vi "DOCK_REPORT_CBATCH_listbox_set_values_and_recolor.vi"(7 "column_names":string[](array[string]), 8 "error_in":errorcluster, 11 "REPORT_all_info_in":T1) -> (0 "error_out":errorcluster, 3 "REPORT_all_info_out":T1)   [LabVIEW 2019]
uses:
  FGV/DOCK_REPORT_records_display/DOCK_REPORT_all_info.ctl
  SQL_CLIENT/MAIN/REPORTS/DATES/typedef/REPORT_DATES_statuses.ctl
  FGV/DOCK_REPORT_records_display/DOCK_REPORT_references.ctl
  <vilib>/Utility/miscctls.llb/LVRowAndColumnTypeDef.ctl
  <vilib>/Utility/miscctls.llb/LVRowAndColumnUnsignedTypeDef.ctl
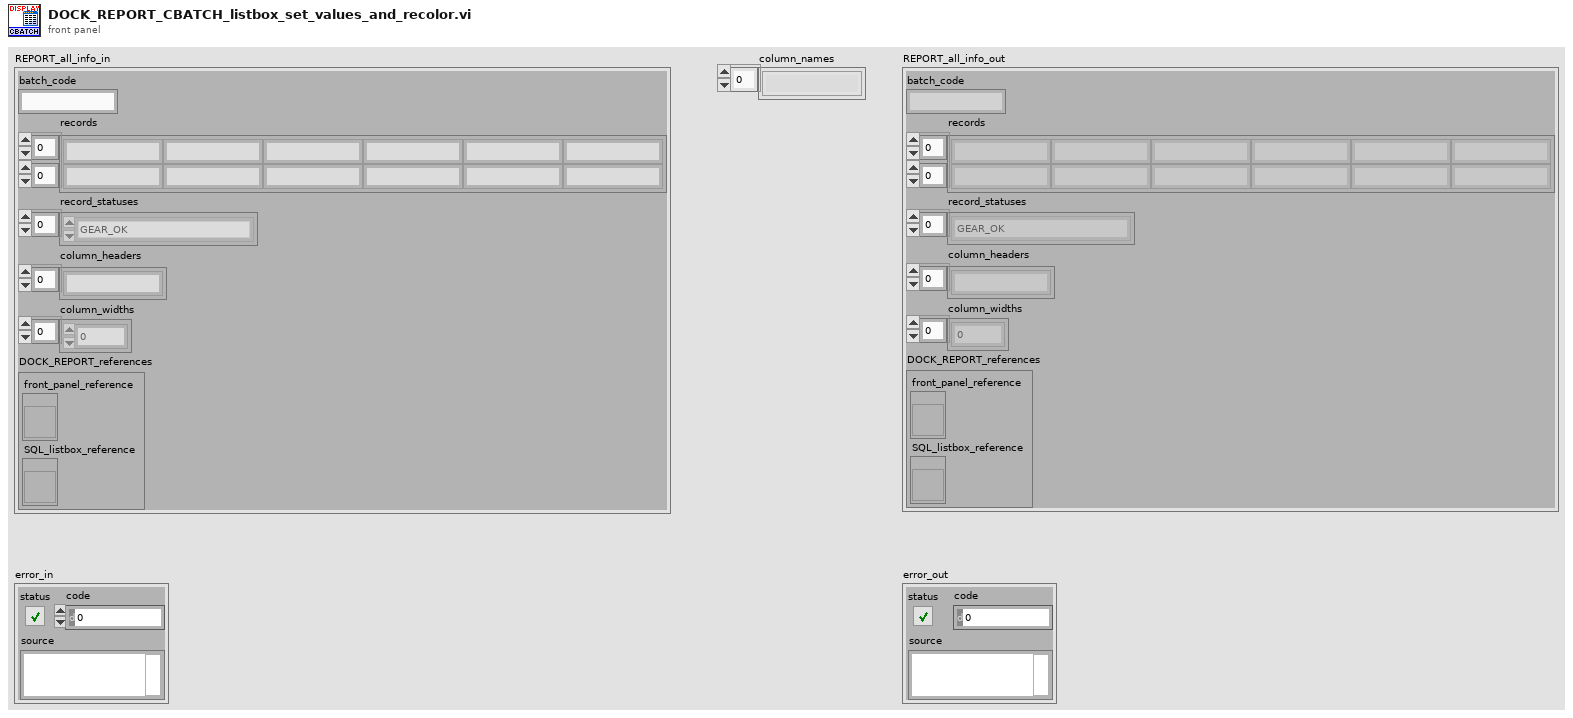
[diagram p1: front panel]
types:
  T1 = typedef "DOCK_REPORT_all_info.ctl" = cluster{"batch_code":string, "records":string[][], "record_statuses":T2[], "column_headers":string[], "column_widths":i16[], "DOCK_REPORT_references":T3}
  T2 = typedef "REPORT_DATES_statuses.ctl" = enum16{"GEAR_OK", "GEAR_NOK", "GEAR_interrupted", "GEAR_in_operation", "GEAR_unexpected"}
  T3 = typedef "DOCK_REPORT_references.ctl" = cluster{"front_panel_reference":refnum<vi>, "SQL_listbox_reference":refnum<vi>}
  T4 = typedef "LVRowAndColumnUnsignedTypeDef.ctl" = cluster{"Row":u32, "Column":u32}
  T5 = typedef "LVRowAndColumnTypeDef.ctl" = cluster{"Row":i32, "Column":i32}
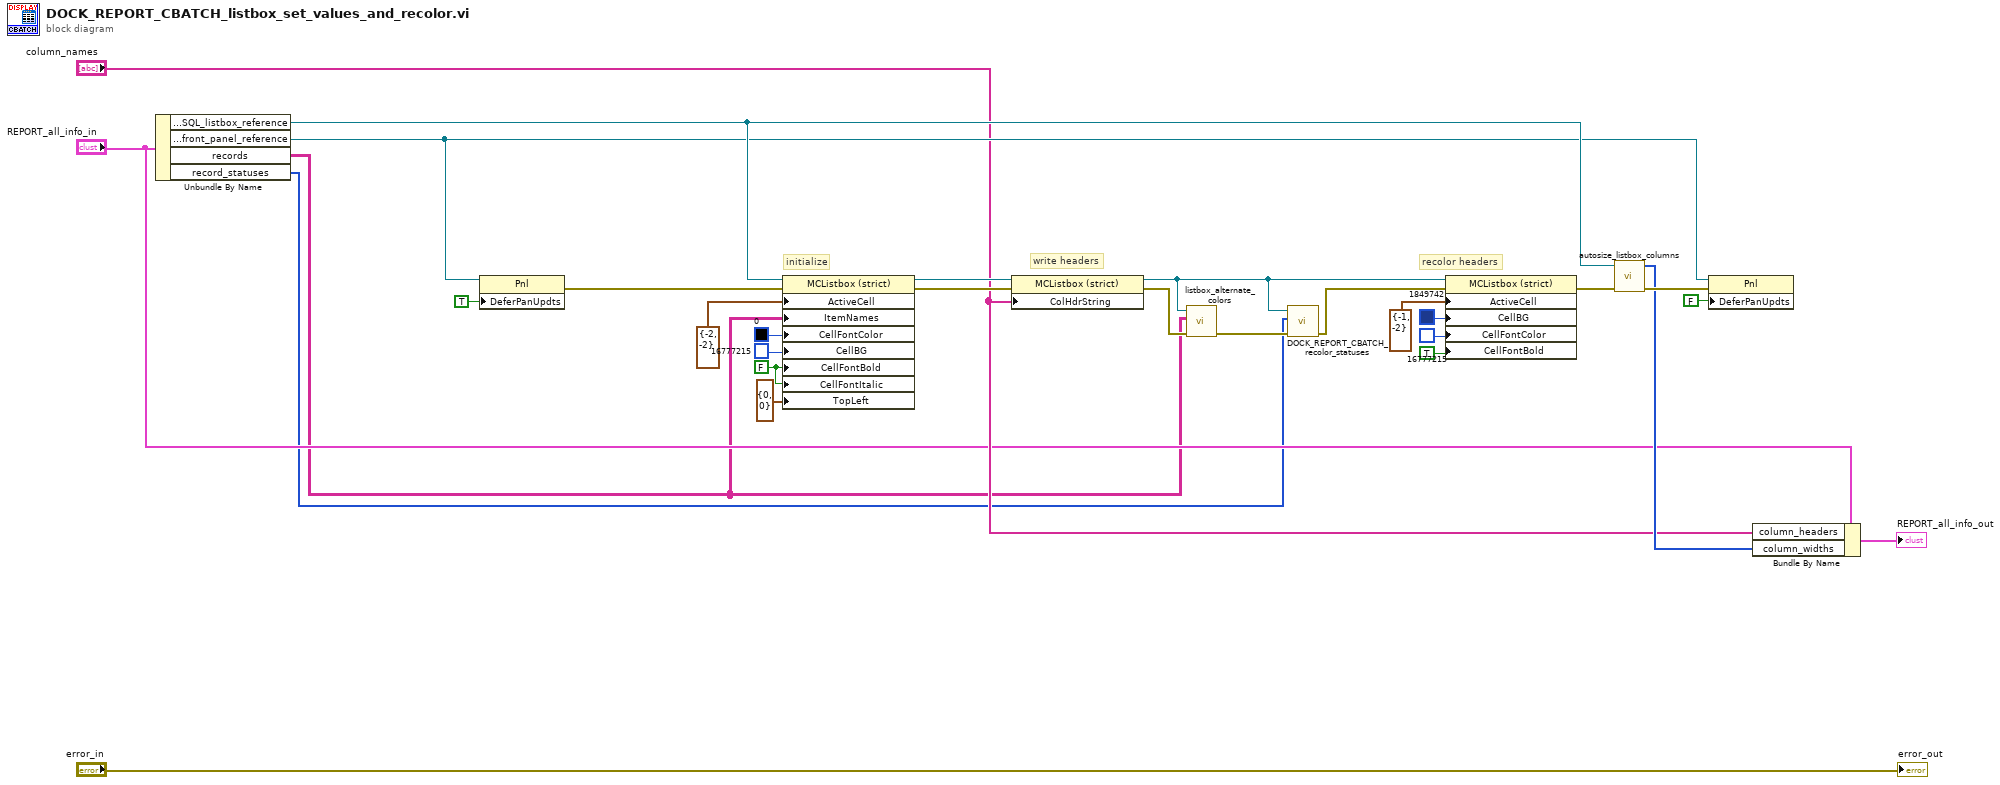
[diagram p0: block diagram]
diagram:
  w19 = FALSE ("Active Cell:Cell Font:Bold")
  # "recolor headers"
  # "initialize"
  # "write headers"
  n1 = Unbundle By Name("REPORT_all_info_in") -> ("DOCK_REPORT_references.SQL_listbox_reference"=w22:refnum<vi>, "DOCK_REPORT_references.front_panel_reference"=w21:refnum<vi>, "records"=w3:string[][], "record_statuses"=w2:T2[])
  n2 = property on="Property Node" class="Pnl"(reference=w21, "DeferPanUpdts"=TRUE ("Defer Panel Updates")) -> (error out=w5:errorcluster)  [unwired: 1 in, 1 out]
  n3 = property on="Property Node" class="MCListbox (strict)"(reference=w22, error in=w5, "ActiveCell"=T5 {"Row"=-2, "Column"=-2} ("Active Cell:Active Cell"), "ItemNames"=w3, "CellFontColor"=u32 0, "CellBG"=u32 16777215, "CellFontBold"=w19, "CellFontItalic"=w19, "TopLeft"=T4 {"Row"=0, "Column"=0} ("Top Left Visible Cell")) -> (reference out=w25:refnum<vi>, error out=w23:errorcluster)
  n4 = property on="Property Node" class="MCListbox (strict)"(reference=w25, error in=w23, "ColHdrString"="column_names") -> (reference out=w12:refnum<vi>, error out=w10:errorcluster)
  n5 = call "listbox_alternate_colors.vi"("error_in"=w10, "item_names"=w3, "listbox_ref"=w12) -> ("error_out"=w11:errorcluster)  [unwired: 8 in]
  n6 = call "DOCK_REPORT_CBATCH_recolor_statuses.vi"("error_in"=w11, "record_statuses"=w2, "listbox_ref"=w12) -> ("error_out"=w9:errorcluster)  [unwired: 8 in]
  n7 = property on="Property Node" class="MCListbox (strict)"(reference=w12, error in=w9, "ActiveCell"=T5 {"Row"=-1, "Column"=-2} ("Active Cell:Active Cell"), "CellBG"=u32 1849742, "CellFontColor"=u32 16777215, "CellFontBold"=TRUE ("Active Cell:Cell Font:Bold")) -> (error out=w27:errorcluster)  [unwired: 1 out]
  n8 = call "autosize_listbox_columns.vi"("error in (no error)"=w27, "Table Ref"=w22) -> ("error out"=w26:errorcluster, "column_widths"=w7:i16[])  [unwired: 4 in]
  n9 = property on="Property Node" class="Pnl"(reference=w21, error in=w26, "DeferPanUpdts"=FALSE ("Defer Panel Updates")) -> ()  [unwired: 2 out]
  n10 = Bundle By Name(cluster="REPORT_all_info_in", "column_headers"="column_names", "column_widths"=w7) -> (→"REPORT_all_info_out":T1)
  "error_out" <- "error_in"
